vi "CheckScanStatus.vi"(8 "error in":T1) -> (0 "error out":T1, 3 "Scanner status":T2(ring))   [LabVIEW 2016]
doc: "This VI returns the scanner status. Distinguished are \"ready\", \"paused\", \"running\", \"adjusting\" and \"returning to origin\"."
uses:
  Controls/Error_Out.ctl
  Files_ASC500/DLL/ASC500_RemoteControlV27.dll
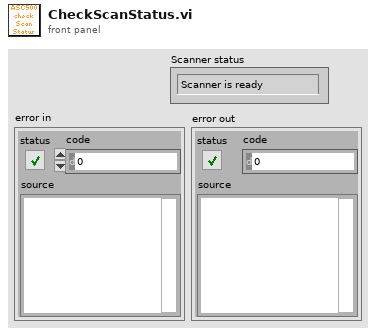
[diagram p1: front panel]
types:
  T1 = typedef "Error_Out.ctl" = errorcluster
  T2 = enum16{"Scanner is ready", "Scanner is running", "Scanner is paused", "Scanner is adjusting", "Scanner is returning to origin"}
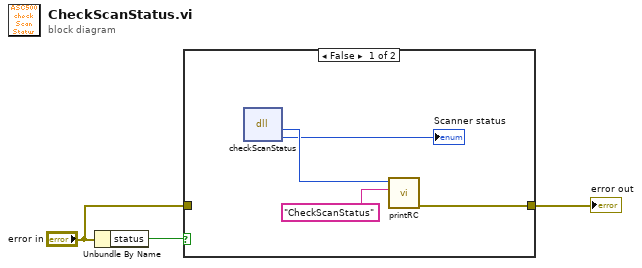
[diagram p0: block diagram]
diagram:
  n1 = Unbundle By Name("error in") -> ("status"=w3:bool)
  n2 = case shown="False" w3 {
    tunnel: "error in" -> [_ w8]
    tunnel: [w4 w8] -> w1
    frame False {
      n3 = dll-call lib="G:/SCMOperations/Share/ELE/Produkt Information/ASC500/04 Remote Control/02 development versions/2018Nov06/Files_ASC500/DLL/ASC500_RemoteControlV27.dll" fn="checkScanStatus"() -> ("RC"=w7:i32, "status"=→"Scanner status":i32)  [unwired: 4 in, 2 out]
      n4 = call "printRC.vi"("additional information"="CheckScanStatus", "RC"=w7) -> ("error out"=w4:T1)  [unwired: 9 in]
    }
    frame True {
    }
  }
  "error out" <- w1
